vi "More_Spreadsheets.vi"() -> ()   [LabVIEW 2020]
uses:
  <vilib>/Utility/file.llb/Write Delimited Spreadsheet (DBL).vi
panel:
  out "Transposed Array":dbl[][](array[numeric]) format="%#_2g"
  out "Generated Array":dbl[][](array[numeric]) format="%#_2g"
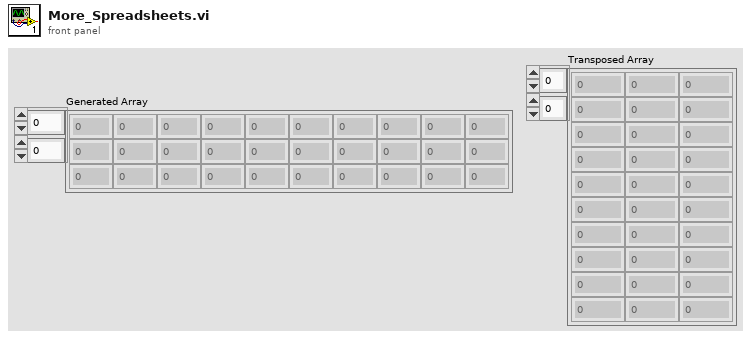
[diagram p1: front panel]
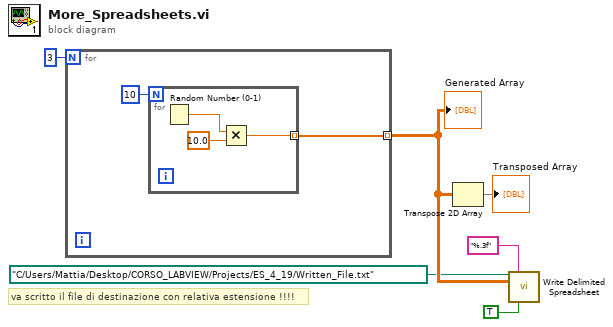
[diagram p0: block diagram]
diagram:
  # "va scritto il file di destinazione con relativa estensione !!!!"
  n1 = for {
    N: 3 -> [_]
    tunnel: [w7] -> w3 mode=indexing
    n2 = for {
      N: 10 -> [_]
      tunnel: [w9] -> w7 mode=indexing
      n3 = Random Number (0-1)() -> (number: 0 to 1=w11:dbl)
      n4 = Multiply(x=w11, y=10.0) -> (x*y=w9:dbl)
    }
  }
  "Generated Array" <- w3
  n5 = Transpose 2D Array(2D array=w3) -> (transposed array=→"Transposed Array":dbl[][])
  n6 = call-poly <vilib>:"Write Delimited Spreadsheet.vi"("file path (dialog if empty)"=path "C:/Users/Mattia/Desktop/CORSO_LABVIEW/Projects/ES_4_19/Written_File.txt", "format (%.3f)"="%.3f", "2D data"=w3, "transpose? (no:F)"=TRUE) -> ()  [unwired: 10 in, 2 out]
